vi "StartClone.vi"(7 "ShowPanel? (f)":bool, 8 "error in (no error)":errorcluster, 10 "ModuleName":string="unnamed", 11 "VI Refnum":refnum<vi>) -> (0 "error out":errorcluster, 1 "clBroadcastEvents":T1, 3 "ModuleAdmin":refnum<class "ModuleAdmin.lvclass">)   [LabVIEW 2014, in "ScopeModule.lvlib"]
uses:
  ScopeModule.lvlib
  Protected/Broadcasts/clBroadcastEvents.ctl
  Protected/clEventType.ctl
  <userlib>/NIST/ModuleAdminLib/ModuleAdmin/ModuleAdmin.lvclass
  <userlib>/NIST/ModuleAdminLib/CloneRegistration/CloneRegistration.lvclass
  <userlib>/NIST/ModuleAdminLib/ModuleAdmin/ModuleAdmin.lvclass/ModuleAdmin.ctl
  <userlib>/NIST/ModuleAdminLib/ModuleAdmin/Accessors/Write CloneRegRef.vi
  <userlib>/NIST/ModuleAdminLib/ModuleAdmin/Accessors/Write ShowPanel_.vi
  <vilib>/Utility/error.llb/Error Cluster From Error Code.vi
  <vilib>/ErrorRing/Error Ring.xnode
  <userlib>/NIST/ModuleAdminLib/ModuleAdminBase/ModuleAdminBase.lvclass
panel:
  # "If you want to add other Broadcast Events, open this typedef, copy an existing event and rename it to your event name.\n\nNext create an \"arg\" typedef for the  data and put it into PublicAPI/Arguments/Broadcasts\n\nAfter that, you will need to create a new roadcast vi in Protected/Broadcast.  Look at DidInit.vi or the reportError.vi as examples."
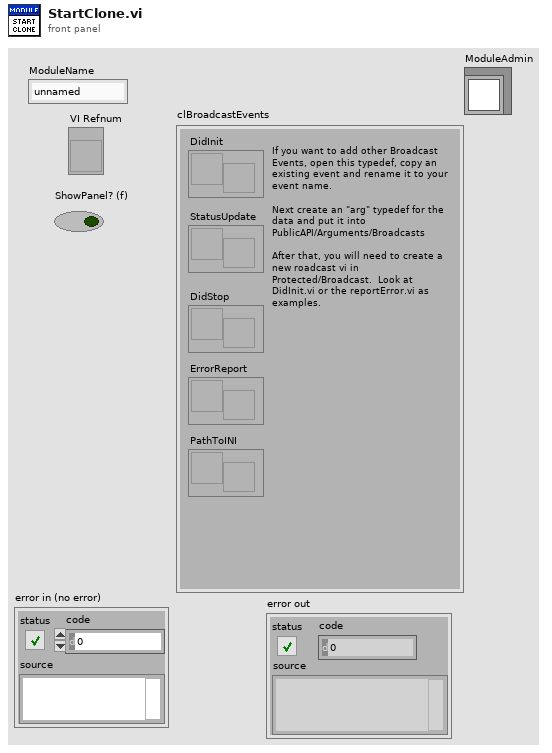
[diagram p1: front panel]
types:
  T1 = typedef "ScopeModule.lvlib/clBroadcastEvents.ctl" = cluster{"DidInit":refnum<user-event>, "StatusUpdate":refnum<user-event>, "ErrorReport":refnum<user-event>, "DidStop":refnum<user-event>, "PathToINI":refnum<user-event>}
  T2 = enum32{"Bad", "Idle", "Run top level", "Running"}
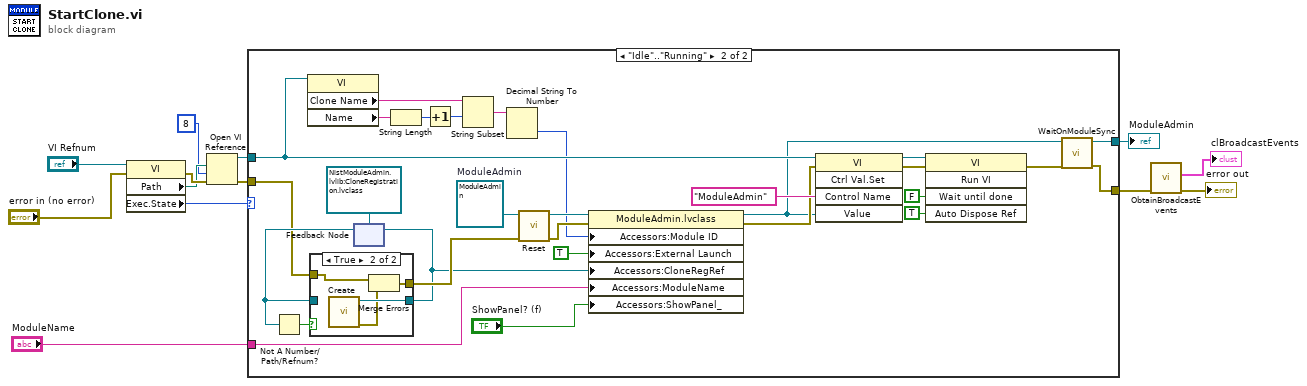
[diagram p0: block diagram]
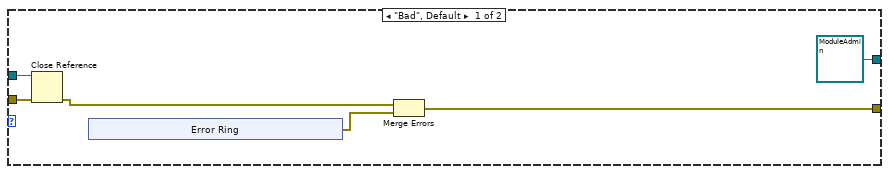
[diagram p2: hidden frame]
diagram:
  n1 = property class="VI"(reference="VI Refnum", error in="error in (no error)") -> (error out=w11:errorcluster, "Path"=w10:path, "Exec.State"=w12:T2)  [unwired: 1 out]
  n2 = Open VI Reference(vi path=w10, options=8, error in (no error)=w11) -> (vi reference=w8:refnum<vi>, error out=w9:errorcluster)  [unwired: 3 in]
  n3 = case shown="\"Idle\"..\"Running\"" w12 {
    tunnel: w9 -> [w19 w28]
    tunnel: w8 -> [w18 w43]
    tunnel: [w15 w33] -> w5
    tunnel: "ModuleName" -> [_ w32]
    tunnel: [refnum<class "ModuleAdmin.lvclass"> refnum ("ModuleAdmin") w25] -> w1
    frame "Bad", Default {
      n4 = Close Reference(reference=w18, error in (no error)=w19) -> (error out=w17:errorcluster)
      n5 = xnode "Error Ring"() -> ("error out"=w16:errorcluster)
      n6 = Merge Errors(w17, w16) -> (w15:errorcluster)
    }
    frame "Idle".."Running" {
      w47 = refnum<class "ModuleAdmin.lvclass"> refnum  # ModuleAdmin
      n7 = property class="VI"(reference=w43) -> ("Clone Name"=w49:string, "Name"=w52:string)  [unwired: 1 in, 2 out]
      n8 = feedback #1(refnum<data-value> refnum ("CloneRegRef")) -> (w31:refnum<data-value>)
      n9 = Not A Number/Path/Refnum?(number/path/refnum=w31) -> (NaN/Path/Refnum?=w30:bool)
      n10 = case shown="True" w30 {
        tunnel: [w54 w58] -> w26
        tunnel: w31 -> [w54 _]
        tunnel: w28 -> [w53 w56]
        tunnel: [w53 w55] -> w27
        frame False {
        }
        frame True {
          n11 = call <userlib>:"Create.vi"() -> ("error out"=w57:errorcluster, "CloneRegRef"=w58:refnum<data-value>)  [unwired: 10 in]
          n12 = Merge Errors(w56, w57) -> (w55:errorcluster)
        }
      }
      n13 = feedback-in #1(w26) -> ()
      n14 = String Length(string=w52) -> (length=w51:i32)
      n15 = Increment(x=w51) -> (x+1=w50:i32)
      n16 = String Subset(string=w49, offset (0)=w50) -> (substring=w48:string)  [unwired: 1 in]
      n17 = Decimal String To Number(string=w48) -> (number=w35:i32)  [unwired: 2 in, 1 out]
      n18 = call <userlib>:"Reset.vi"("error in (no error)"=w27, "Mod Admin in"=w47) -> ("error out"=w46:errorcluster, "Mod Admin out"=w45:refnum<class "ModuleAdmin.lvclass">)  [unwired: 8 in]
      n19 = property class="ModuleAdmin.lvclass"(reference=w45, error in=w46, "Accessors:Module ID"=w35, "Accessors:External Launch"=TRUE ("External Launch"), "Accessors:CloneRegRef"=w26, "Accessors:ModuleName"=w32, "Accessors:ShowPanel_"="ShowPanel? (f)") -> (reference out=w34:refnum<class "ModuleAdmin.lvclass">, error out=w36:errorcluster)
      n20 = invoke class="VI" method="Ctrl Val.Set"(reference=w43, error in=w36, "Control Name"="ModuleAdmin", "Value"=w34) -> (reference out=w41:refnum<vi>, error out=w40:errorcluster)  [unwired: 1 in, 3 out]
      n21 = invoke class="VI" method="Run VI"(reference=w41, error in=w40, "Wait until done"=FALSE ("Wait Until Done"), "Auto Dispose Ref"=TRUE ("Auto Dispose Reference")) -> (error out=w37:errorcluster)  [unwired: 1 in, 4 out]
      n22 = call <userlib>:"WaitOnModuleSync.vi"("error in (no error)"=w37, "ModuleAdmin"=w34) -> ("error out"=w33:errorcluster, "ModuleAdmin"=w25:refnum<class "ModuleAdmin.lvclass">)  [unwired: 8 in]
    }
  }
  "ModuleAdmin" <- w1
  n23 = call "ObtainBroadcastEvents.vi"("error in (no error)"=w5) -> ("error out"=→"error out":errorcluster, "clBroadcastEvents"=→"clBroadcastEvents":T1)  [unwired: 9 in]
